vi "DataTranslation_server.vi"(0 "Board type":T1=enum."DT LV-link", 1 "interval scanning":bool, 2 "Client Time":dbl=3399992102.447224, 5 "No of samples+extra":i32=200 min=0 step=1, 7 "Trigger mode":T2, 9 "output polarity":u16(ring)=1 items=["do not change", "positive", "negative"], 11 "Ch & spans":T3[](array[typedef])=[{"high limit (10V)"=10.0, "low limit (-10V)"=-10.0, "Ch No"=0, "Var name"="RV (Vin)", "Use Latest Calib"=FALSE}] {"low limit (-10V)" format="%.3f"; "high limit (10V)" format="%.3f"}, 12 "Actual Sampling rate (Hz)":dbl=10000.0 format="%.2f", 13 "Local Client?":bool=TRUE, 14 "Current Block No":i32) -> (4 "I16 data":i16[][](array[numeric]), 6 "Block Timings":T4={"Started"=3399991568.753699, "Ended"=3399991587.0837474, "Analogue Frequency Hz"=50000.0} {"Analogue Frequency Hz" format="%.2f"}, 10 "group channel settings":T5(array[cluster])=[{"channel"="", "upper input limits"=0.0, "lower input limits"=0.0, "range"=0.0, "polarity"=0, "gain"=0.0, "coupling"=0, "input mode"=0, "scale multiplier"=1.6666666666666668e-07, "scale offset"=0.0}] {"scale offset" format="%#_16f"; "scale multiplier" format="%#_16f"; "input mode" format="%#_16f"; "coupling" format="%#_16f"; "gain" format="%#_16f"; "polarity" format="%#_16f"; "range" format="%#_16f"; "lower input limits" format="%#_16f"; "upper input limits" format="%#_16f"}, 15 "error out":errorcluster={"status"=TRUE, "code"=1172, "source"="Error calling method LvLink2.LvTask.ReadDblData2DAs1D, (System.Reflection.TargetInvocationException: Exception has been thrown by the target of an invocation.\n\tInner Exception: LvLink2.LvException: Timeout) <append><b>LvLink2.LvException</b> in OLReadMultiple2D.vi->DataTranslation_server.vi->Acquire_Data.vi->Get_data.vi->Measurement.vi"})   [LabVIEW 2011]
uses:
  Controls/Block_start_and_end.ctl
  Data_Translation/DataTranslation_global.vi
  Globals/Meas_global.vi
  <userlib>/LV-Link3/PolySubVIs/DtCreateAinChan.vi
  PWA/PWAtasksGLOBAL.vi
  <userlib>/LV-Link3/PolySubVIs/DtOLTimingSetInput.vi
  <userlib>/LV-Link3/PolySubVIs/DtOLReadMultiple2D.vi
  <userlib>/LV-Link3/PolySubVIs/DtOLTriggerDigital.vi
  Controls/Ch_and_Spans.ctl
  Controls/Trigger_Mode.ctl
  Controls/Board_Types.ctl
panel:
  in  "error in":errorcluster
  out "AFG error out":errorcluster
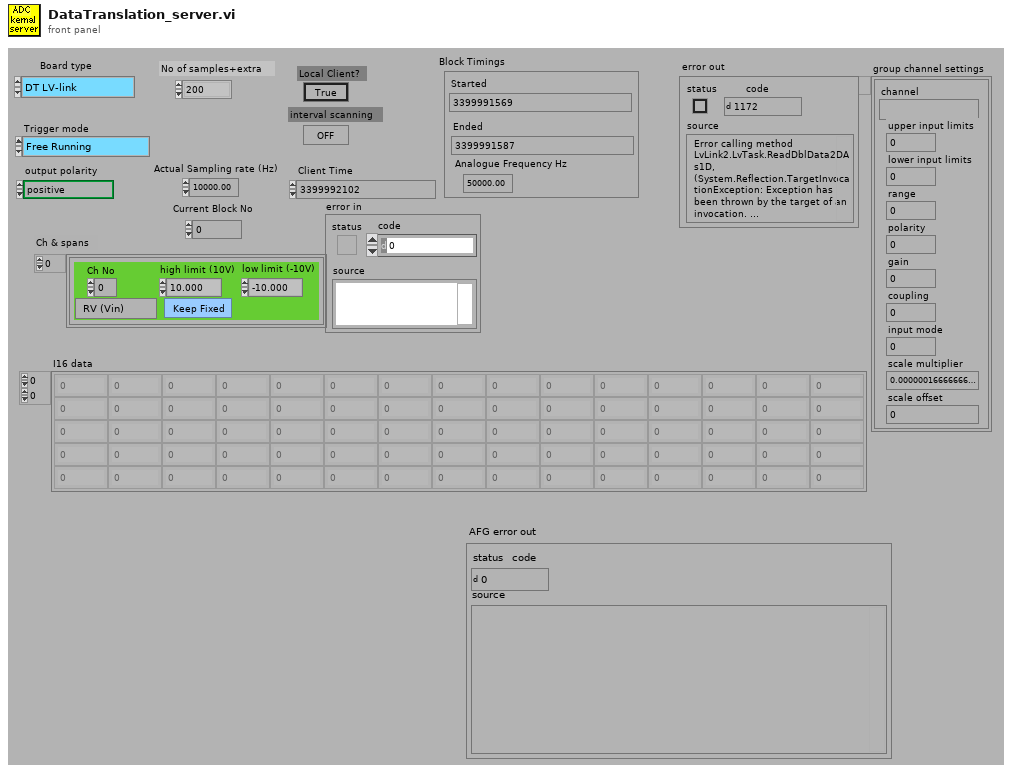
[diagram p1: front panel]
types:
  T1 = typedef "Board_Types.ctl" = enum16{"Simulate", "Local ADAM", "Server ADAM", "NI-DAQmx", "NI-DAQmxBase", "ADC488", "DT LV-link"}
  T2 = typedef "Trigger_Mode.ctl" = enum16{"Free Running", "Start on Trigger", "Trigger Every Block", "Trigger Every Sample"}
  T3 = typedef "Ch_and_Spans.ctl" = cluster{"high limit (10V)":sgl, "low limit (-10V)":sgl, "Ch No":i16, "Var name":string, "Use Latest Calib":bool}
  T4 = typedef "Block_start_and_end.ctl" = cluster{"Started":dbl, "Ended":dbl, "Analogue Frequency Hz":dbl}
  T5 = cluster{"channel":string, "upper input limits":sgl, "lower input limits":sgl, "range":sgl, "polarity":u16, "gain":sgl, "coupling":u16, "input mode":u16, "scale multiplier":dbl, "scale offset":dbl}[]
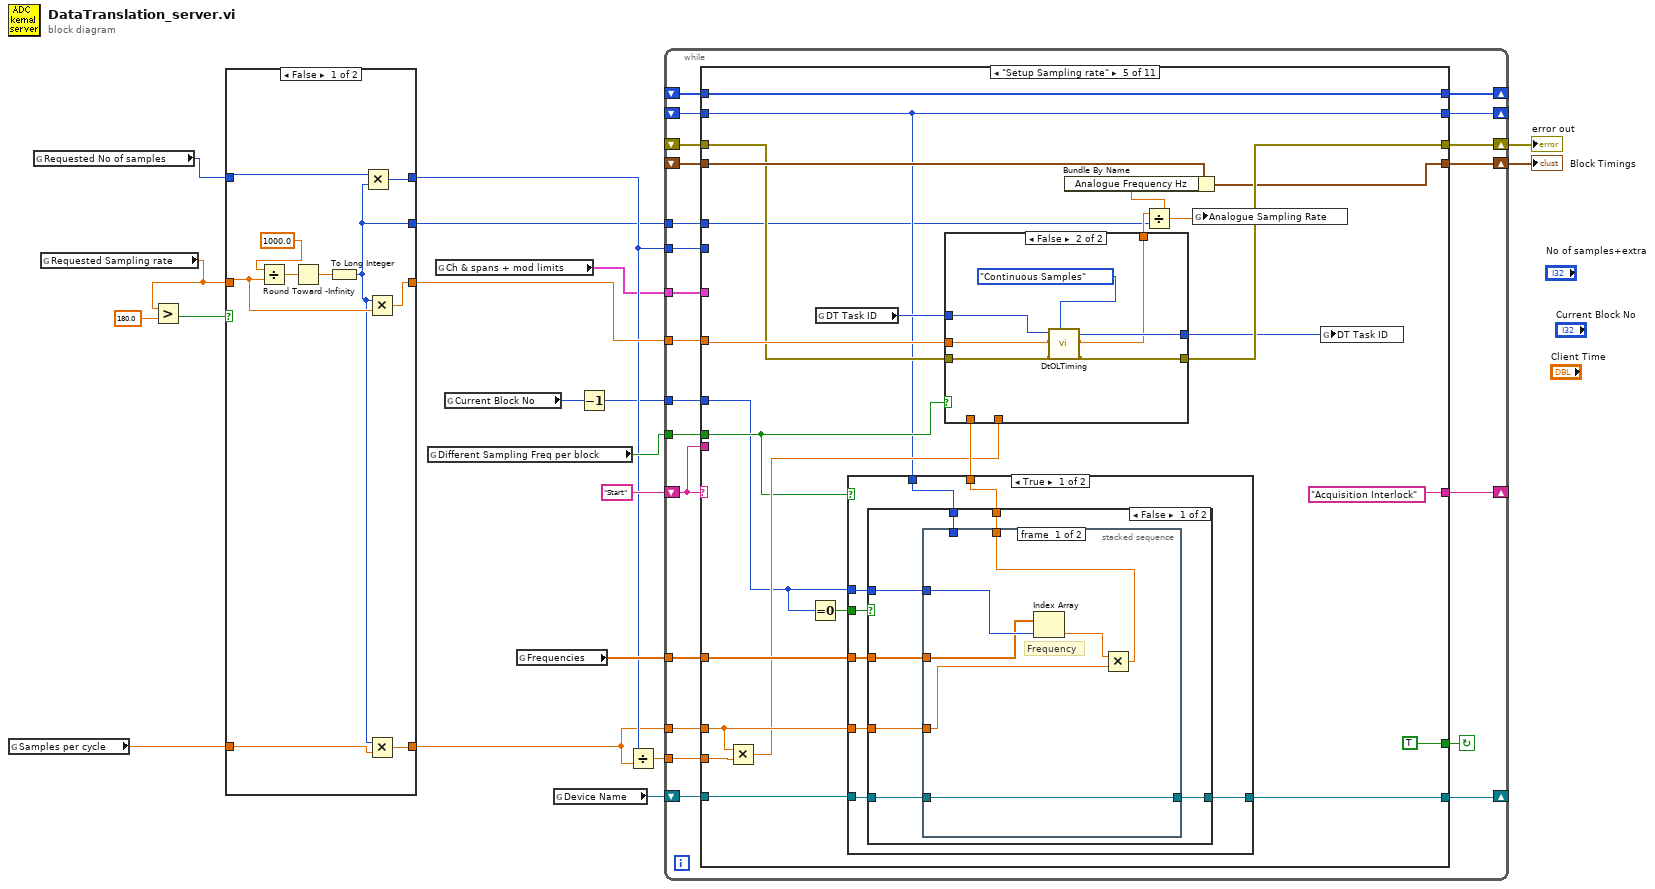
[diagram p0: block diagram]
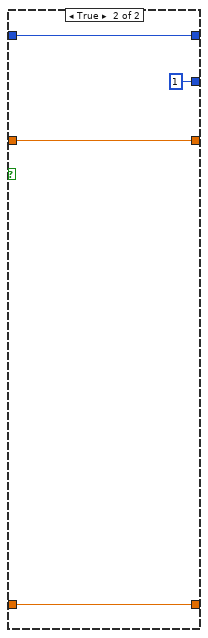
[diagram p2: hidden frame]
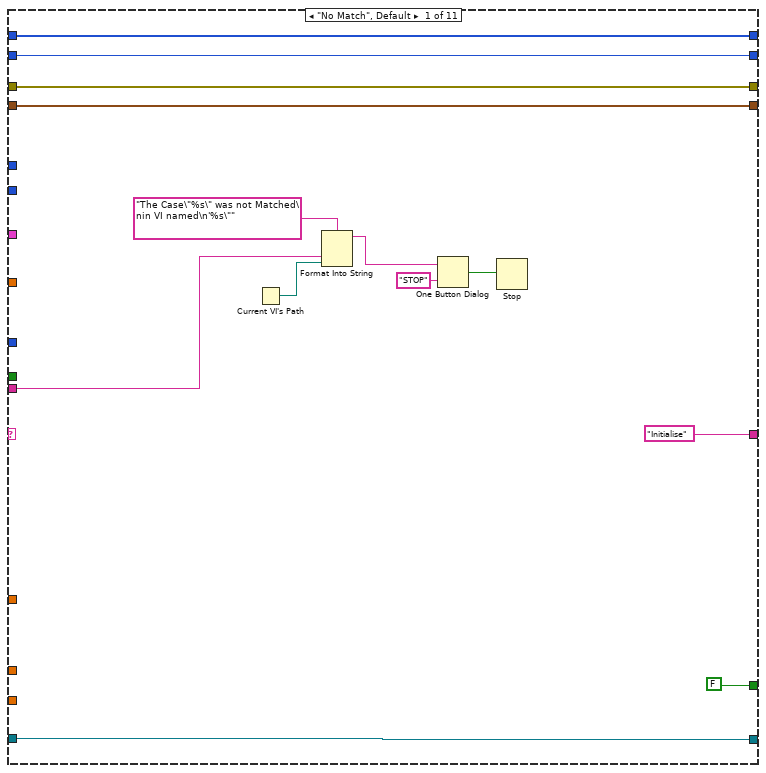
[diagram p3: hidden frame]
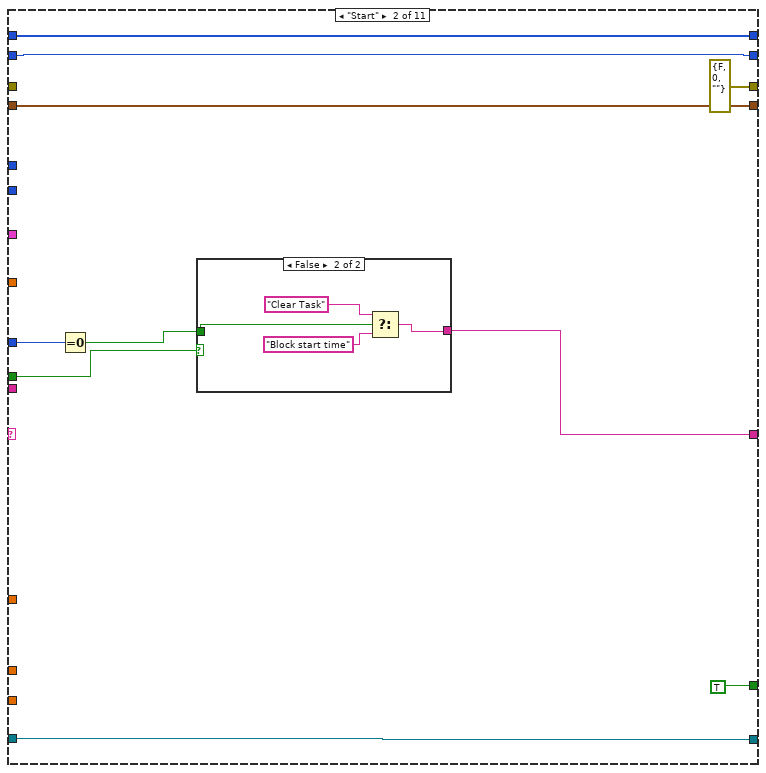
[diagram p4: hidden frame]
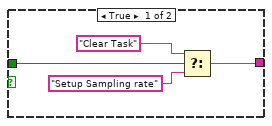
[diagram p5: hidden frame]
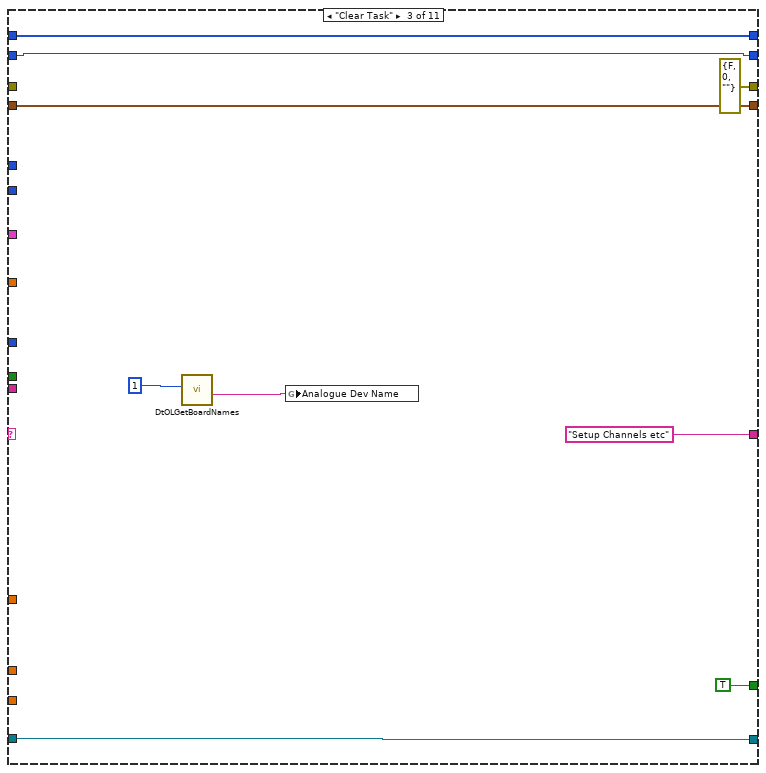
[diagram p6: hidden frame]
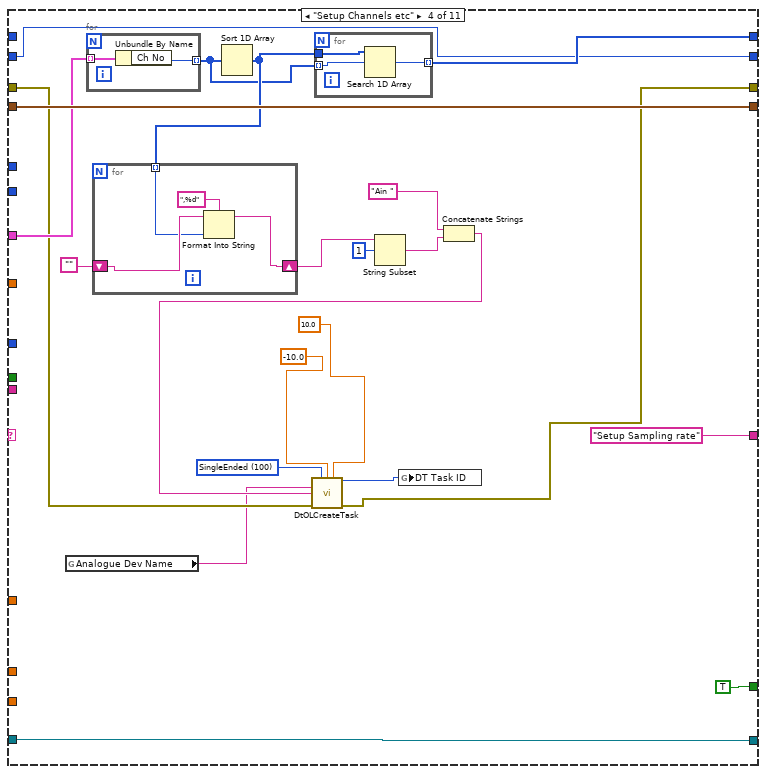
[diagram p7: hidden frame]
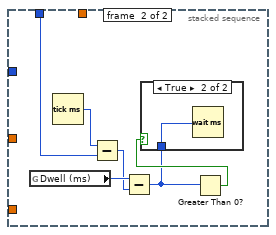
[diagram p8: hidden frame]
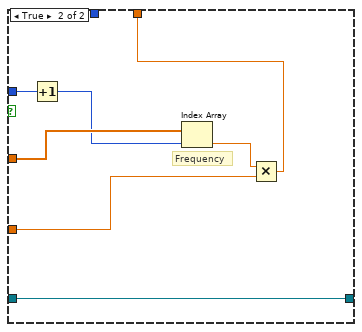
[diagram p10: hidden frame]
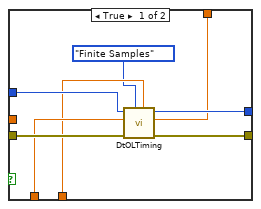
[diagram p12: hidden frame]
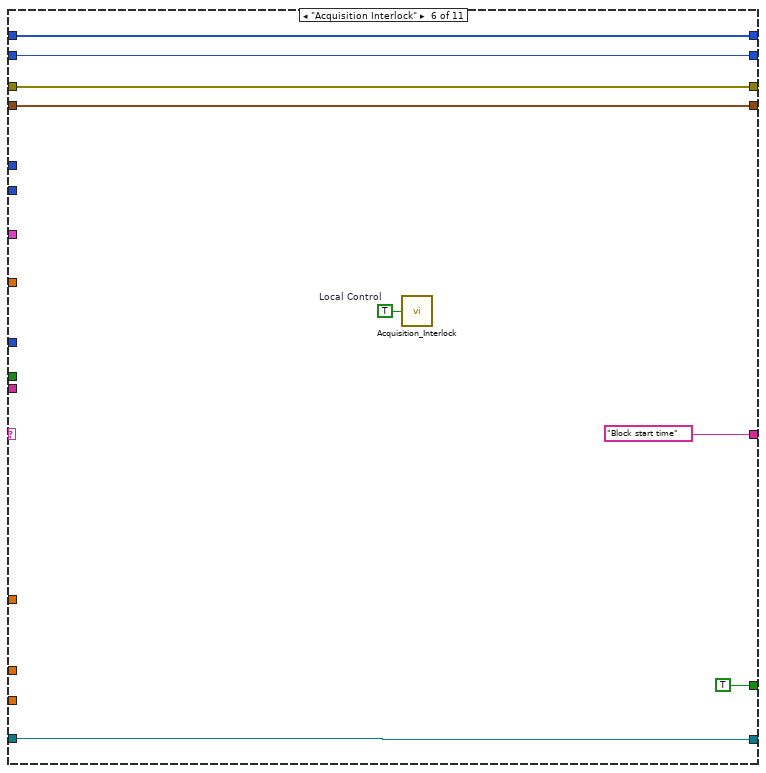
[diagram p13: hidden frame]
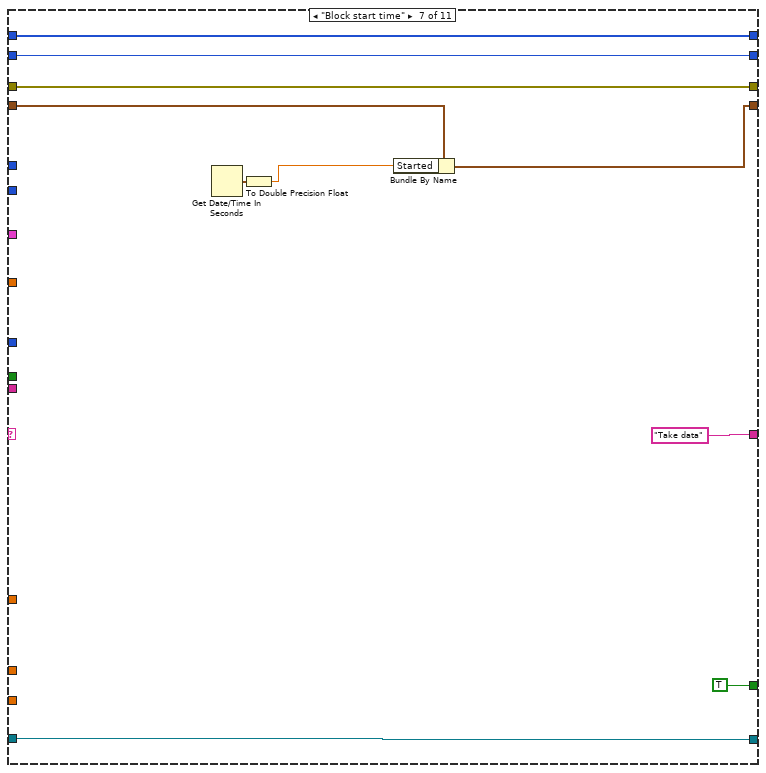
[diagram p14: hidden frame]
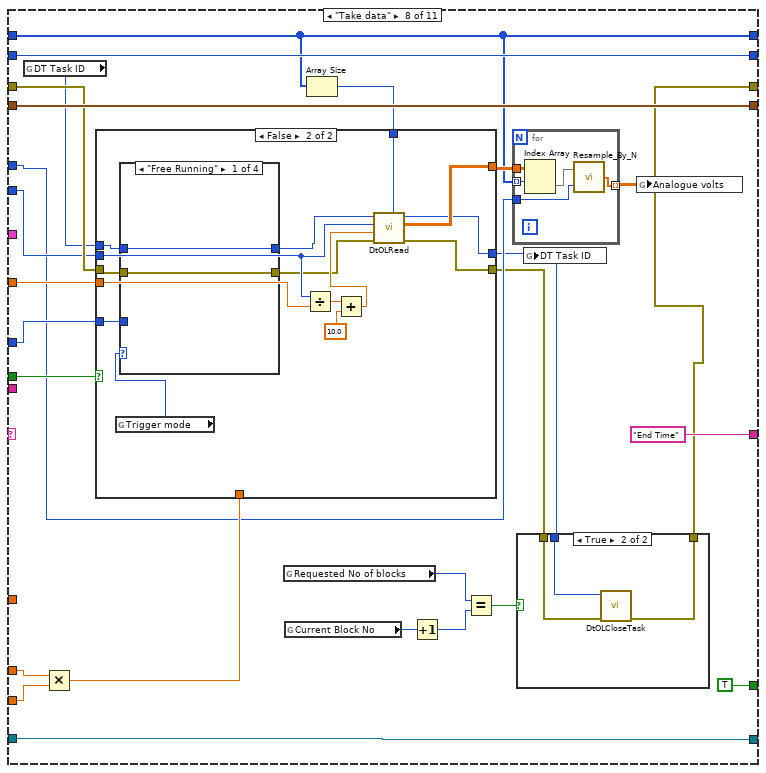
[diagram p15: hidden frame]
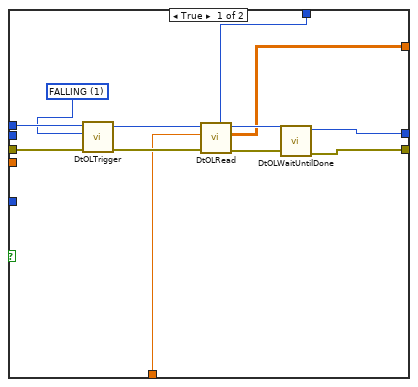
[diagram p17: hidden frame]
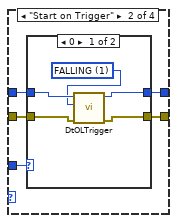
[diagram p18: hidden frame]
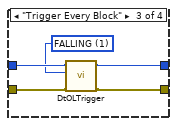
[diagram p20: hidden frame]
diagram:
  n1 = global read "DataTranslation_global.vi" "Samples per cycle"() -> (w7:dbl)
  n2 = global read "Meas_global.vi" "Requested No of samples"() -> (w1:i32)
  n3 = global read "Meas_global.vi" "Requested Sampling rate"() -> (w4:dbl)
  n4 = Greater?(x=w4, y=180.0) -> (0:w11:bool)
  n5 = case shown="False" w11 {
    tunnel: w4 -> [w23 w33]
    tunnel: [w24 w33] -> w10
    tunnel: [w26 w32] -> w9
    tunnel: w1 -> [w25 w32]
    tunnel: [w22 w31] -> w8
    tunnel: w7 -> [w21 w31]
    tunnel: [w20 1] -> w6
    frame False {
      n6 = Divide(x=1000.0, y=w23) -> (x/y=w28:dbl)
      n7 = Round Toward -Infinity(1:w28) -> (0:w27:dbl)
      n8 = To Long Integer(number=w27) -> (32bit integer=w20:i32)
      n9 = Multiply(x=w25, y=w20) -> (x*y=w26:i32)
      n10 = Multiply(x=w20, y=w23) -> (x*y=w24:dbl)
      n11 = Multiply(x=w20, y=w21) -> (x*y=w22:dbl)
    }
    frame True {
    }
  }
  n12 = global read "DataTranslation_global.vi" "Different Sampling Freq per block"() -> (w13:bool)
  n13 = global read "Meas_global.vi" "Ch & spans + mod limits"() -> (w5:T3[])
  n14 = global read "Meas_global.vi" "Current Block No"() -> (w3:i32)
  n15 = global read "DataTranslation_global.vi" "Frequencies"() -> (w14:dbl[])
  n16 = global read "DataTranslation_global.vi" "Device Name"() -> (w15:refnum<visa-resource-name>)
  n17 = Decrement(x=w3) -> (x-1=w2:i32)
  n18 = Divide(x=w9, y=w8) -> (x/y=w16:dbl)
  n19 = while {
    shift-left: "Start" -> [w53]
    shift-right: [w54] -> _
    shift-right: [w46] -> w17
    shift-left: _ -> [w52]
    shift-right: [w45] -> w18
    shift-left: _ -> [w51]
    tunnel: w10 -> [w50]
    tunnel: w9 -> [w49]
    tunnel: w2 -> [w48]
    tunnel: w5 -> [w47]
    shift-right: [w44] -> _
    shift-left: _ -> [w43]
    tunnel: w8 -> [w41]
    shift-right: [w40] -> _
    shift-left: w15 -> [w42]
    tunnel: w16 -> [w39]
    tunnel: w13 -> [w38]
    tunnel: w14 -> [w37]
    shift-right: [w36] -> _
    shift-left: _ -> [w35]
    tunnel: w6 -> [w34]
    stop <- w55 continue-if-true
    n20 = case shown="\"Setup Sampling rate\"" w53 {
      tunnel: [FALSE TRUE TRUE TRUE TRUE TRUE TRUE TRUE w307 FALSE FALSE] -> w55
      tunnel: ["Initialise" w74 "Setup Channels etc" "Setup Sampling rate" "Acquisition Interlock" "Block start time" "Take data" "End Time" "Add info to block header" ("f") "End" ("f") "End" ("f")] -> w54
      tunnel: w53 -> [w63 _ _ _ _ _ _ _ _ _ _]
      tunnel: [w60 errorcluster {"status"=FALSE, "code"=0, "source"=""} ("error out") errorcluster {"status"=FALSE, "code"=0, "source"=""} ("error out") w98 w149 w209 w217 w222 w309 w329 w374] -> w46
      tunnel: w52 -> [w60 _ _ w99 w145 w209 w217 w243 w309 w329 w374]
      tunnel: [w59 w77 w94 w110 w146 w207 w218 w244 w311 w327 T4 {"Started"=0.0, "Ended"=0.0, "Analogue Frequency Hz"=1000.0} ("Block Timings")] -> w45
      tunnel: w51 -> [w59 w77 w94 w110 w147 w207 w219 w244 w312 w327 _]
      tunnel: w50 -> [_ _ _ _ w148 _ _ w239 _ _ _]
      tunnel: w49 -> [_ _ _ _ _ _ _ w240 _ _ _]
      tunnel: w48 -> [_ w76 _ _ w131 _ _ w232 _ w317 _]
      tunnel: w47 -> [_ _ _ w109 _ _ _ _ _ _ _]
      tunnel: [w58 w72 w92 w106 w142 w206 w214 w231 w308 w328 w372] -> w44
      tunnel: w43 -> [w58 w72 w92 _ w142 w206 w214 w231 w308 w328 w372]
      tunnel: w42 -> [w57 w71 w91 w105 w139 w205 w213 w238 w306 w326 w371]
      tunnel: w37 -> [_ _ _ _ w141 _ _ _ _ w322 _]
      tunnel: w41 -> [_ _ _ _ w135 _ _ w236 _ _ _]
      tunnel: [w57 w71 w91 w105 w138 w205 w213 w238 w306 w325 w371] -> w40
      tunnel: w39 -> [_ _ _ _ w136 _ _ w237 _ _ _]
      tunnel: w38 -> [_ w70 _ _ w133 _ _ w234 w307 _ _]
      tunnel: [w56 w69 w90 w104 w132 w204 w212 w233 w305 w319 w370] -> w36
      tunnel: w35 -> [w56 w69 w90 w104 w132 w204 w212 w233 w305 _ w370]
      tunnel: w34 -> [_ _ _ _ w128 _ _ w229 _ _ _]
      frame "No Match", Default {
        n21 = Current VI's Path() -> (path=w62:path)
        n22 = Format Into String(format string="The Case\"%s\" was not Matched\nin VI named\n'%s\"" ("Format String"), w63, w62) -> (resulting string=w66:string)  [unwired: 2 in, 1 out]
        n23 = One Button Dialog(message=w66, button name ("OK")="STOP") -> (true=w64:bool)
        n24 = Stop(stop? (T)=w64) -> ()
      }
      frame "Start" {
        n25 = Equal To 0?(x=w76) -> (x = 0?=w75:bool)
        n26 = case shown="False" w70 {
          tunnel: w75 -> [w80 w84]
          tunnel: [w79 w83] -> w74
          frame True {
            n27 = Select(t="Clear Task", s=w80, f="Setup Sampling rate") -> (s? t:f=w79:string)
          }
          frame False {
            n28 = Select(t="Clear Task", s=w84, f="Block start time") -> (s? t:f=w83:string)
          }
        }
      }
      frame "Clear Task" {
        n29 = call <userlib>:"DtOLGetBoardNames.vi"("Select Board"=u32 1) -> ("Board Name"=w88:string)  [unwired: 8 in, 2 out]
        n30 = global write "PWAtasksGLOBAL.vi" "Analogue Dev Name"(w88) -> ()
      }
      frame "Setup Channels etc" {
        w100 = 100 items=["SingleEnded"=100, "Differential"=101] ("Channel Type")
        n31 = global read "PWAtasksGLOBAL.vi" "Analogue Dev Name"() -> (w96:string)
        n32 = for {
          tunnel: w109 -> [w122] mode=indexing
          tunnel: [w121] -> w107 mode=indexing
          n33 = Unbundle By Name(w122) -> ("Ch No"=w121:i16)
        }
        n34 = Sort 1D Array(array=w107) -> (sorted array=w108:i16[])
        n35 = for {
          shift-right: [w124] -> w115
          shift-left: "" -> [w125]
          tunnel: w108 -> [w123] mode=indexing
          n36 = Format Into String(format string=",%d", initial string=w125, w123) -> (resulting string=w124:string)  [unwired: 1 in, 1 out]
        }
        n37 = for {
          tunnel: w108 -> [w120]
          tunnel: w107 -> [w119] mode=indexing
          tunnel: [w118] -> w106 mode=indexing
          n38 = Search 1D Array(1D array=w120, element=w119) -> (index of element=w118:i32)  [unwired: 1 in]
        }
        n39 = String Subset(string=w115, offset (0)=1) -> (substring=w112:string)  [unwired: 1 in]
        n40 = Concatenate Strings("Ain ", w112) -> (w103:string)
        n41 = call-poly <userlib>:"DtOLCreateTask.vi"("Channel Type"=w100, "Range Min"=-10.0, "Range Max"=10.0, "Board Name"=w96, "Channel"=w103, "error in (no error)"=w99) -> ("Task out"=w97:i32, "error out"=w98:errorcluster)  [unwired: 7 in, 1 out]
        n42 = global write "DataTranslation_global.vi" "DT Task ID"(w97) -> ()
      }
      frame "Setup Sampling rate" {
        n43 = Multiply(x=w135, y=w136) -> (x*y=w134:dbl)
        n44 = Equal To 0?(x=w131) -> (x = 0?=w130:bool)
        n45 = global read "DataTranslation_global.vi" "DT Task ID"() -> (w143:i32)
        n46 = case shown="True" w133 {
          tunnel: w141 -> [w154 _]
          tunnel: [w158 w186] -> w140
          tunnel: w135 -> [w157 w186]
          tunnel: w131 -> [w156 _]
          tunnel: w139 -> [w155 w187]
          tunnel: [w153 w187] -> w138
          tunnel: w132 -> [w152 _]
          tunnel: w130 -> [w151 _]
          frame True {
            n47 = case shown="False" w151 {
              tunnel: [w165 w182] -> w158
              tunnel: w157 -> [w164 w181]
              tunnel: w156 -> [w159 w183]
              tunnel: w155 -> [w163 w180]
              tunnel: w154 -> [w162 w184]
              tunnel: [w161 w180] -> w153
              tunnel: w152 -> [w160 _]
              frame False {
                n48 = stacked-sequence {
                  tunnel: [w171 _] -> w165
                  tunnel: w164 -> [w170 _]
                  tunnel: w159 -> [w169 _]
                  tunnel: w163 -> [w166 _]
                  tunnel: w162 -> [w168 _]
                  tunnel: [w166 _] -> w161
                  tunnel: w160 -> [_ w176]
                  frame #0 {
                    # "Frequency"
                    n49 = Index Array(array=w168, index=w169) -> (element=w167:dbl)
                    n50 = Multiply(x=w167, y=w170) -> (x*y=w171:dbl)
                  }
                  frame #1 {
                    n51 = global read "DataTranslation_global.vi" "Dwell (ms)"() -> (w175:u32)
                    n52 = Tick Count (ms)() -> (millisecond timer value=w177:u32)
                    n53 = Subtract(x=w177, y=w176) -> (x-y=w174:u32)
                    n54 = Subtract(x=w175, y=w174) -> (x-y=w172:u32)
                    n55 = Greater Than 0?(x=w172) -> (x > 0?=w173:bool)
                    n56 = case shown="True" w173 {
                      tunnel: w172 -> [_ w178]
                      frame False {
                      }
                      frame True {
                        n57 = Wait (ms)(milliseconds to wait=w178) -> ()  [unwired: 1 out]
                      }
                    }
                  }
                }
              }
              frame True {
                # "Frequency"
                n58 = Increment(x=w183) -> (x+1=w179:i32)
                n59 = Index Array(array=w184, index=w179) -> (element=w185:dbl)
                n60 = Multiply(x=w185, y=w181) -> (x*y=w182:dbl)
              }
            }
          }
          frame False {
          }
        }
        n61 = case shown="False" w133 {
          tunnel: [w192 w197] -> w149
          tunnel: w148 -> [_ w200]
          tunnel: [w191 w199] -> w129
          tunnel: w145 -> [w193 w198]
          tunnel: [w194 w202] -> w144
          tunnel: w143 -> [w195 w201]
          tunnel: w140 -> [w190 _]
          tunnel: w134 -> [w189 _]
          frame True {
            n62 = call-poly <userlib>:"DtOLTiming.vi"("Samples Per Channel"=w189, "Sample Mode"=enum16{"Finite Samples", "Continuous Samples"}."Finite Samples", "error in (no error)"=w193, "Sample Freq (Hz)"=w190, "Task in"=w195) -> ("error out"=w192:errorcluster, "Actual Sample Freq"=w191:dbl, "Task out"=w194:i32)  [unwired: 3 in, 1 out]
          }
          frame False {
            n63 = call-poly <userlib>:"DtOLTiming.vi"("Sample Mode"=enum16{"Finite Samples", "Continuous Samples"}."Continuous Samples", "error in (no error)"=w198, "Sample Freq (Hz)"=w200, "Task in"=w201) -> ("error out"=w197:errorcluster, "Actual Sample Freq"=w199:dbl, "Task out"=w202:i32)  [unwired: 4 in, 1 out]
          }
        }
        n64 = Divide(x=w129, y=w128) -> (x/y=w127:dbl)
        n65 = Bundle By Name(cluster=w147, "Analogue Frequency Hz"=w127) -> (w146:T4)
        n66 = global write "Meas_global.vi" "Analogue Sampling Rate"(w127) -> ()
        n67 = global write "DataTranslation_global.vi" "DT Task ID"(w144) -> ()
      }
      frame "Acquisition Interlock" {
        w203 = TRUE  # Local Control
        n68 = call "Acquisition_Interlock.vi"("Local Control"=w203) -> ()
      }
      frame "Block start time" {
        n69 = Get Date/Time In Seconds() -> (seconds since 1Jan1904=w220:timestamp)
        n70 = To Double Precision Float(number=w220) -> (double precision float=w211:dbl)
        n71 = Bundle By Name(cluster=w219, "Started"=w211) -> (w218:T4)
      }
      frame "Take data" {
        n72 = global read "DataTranslation_global.vi" "DT Task ID"() -> (w242:i32)
        n73 = Multiply(x=w236, y=w237) -> (x*y=w235:dbl)
        n74 = global read "Meas_global.vi" "Requested No of blocks"() -> (w226:i32)
        n75 = global read "Meas_global.vi" "Current Block No"() -> (w228:i32)
        n76 = Array Size(array=w231) -> (size(s)=w230:i32)
        n77 = case shown="False" w234 {
          tunnel: w243 -> [w262 w272]
          tunnel: [w259 w266] -> w223
          tunnel: [w256 w264] -> w225
          tunnel: w242 -> [w255 w273]
          tunnel: [w253 w265] -> w241
          tunnel: w240 -> [_ w269]
          tunnel: w239 -> [_ w277]
          tunnel: w235 -> [w252 _]
          tunnel: w232 -> [_ w271]
          tunnel: w230 -> [w251 w263]
          frame True {
            w254 = 1 items=["RISING", "FALLING"] ("External Trigger Polarity")
            n78 = call-poly <userlib>:"DtOLTrigger.vi"("error in (no error)"=w262, "External Trigger Polarity"=w254, "Task in"=w255) -> ("error out"=w261:errorcluster, "Task out"=w258:i32)  [unwired: 7 in]
            n79 = call-poly <userlib>:"DtOLRead.vi"("Number Chan to Read"=w251, "error in (no error)"=w261, "Samples Per Channel"=w252, "Task in"=w258) -> ("error out"=w260:errorcluster, "2D Data out"=w253:dbl[][], "Task out"=w257:i32)  [unwired: 3 in, 2 out]
            n80 = call <userlib>:"DtOLWaitUntilDone.vi"("error in"=w260, "Task in"=w257) -> ("error out"=w259:errorcluster, "Task out"=w256:i32)  [unwired: 8 in]
          }
          frame False {
            n81 = global read "Meas_global.vi" "Trigger mode"() -> (w274:T2)
            n82 = case shown="\"Free Running\"" w274 {
              tunnel: [w279 w281 w295 w298] -> w270
              tunnel: w273 -> [w279 w283 w296 w298]
              tunnel: [w278 w280 w292 w297] -> w267
              tunnel: w272 -> [w278 w282 w293 w297]
              tunnel: w271 -> [_ w284 _ _]
              frame "Free Running" {
              }
              frame "Start on Trigger" {
                n83 = case shown="0" w284 {
                  tunnel: w283 -> [w289 w291]
                  tunnel: w282 -> [w287 w290]
                  tunnel: [w285 w291] -> w281
                  tunnel: [w286 w290] -> w280
                  frame 0 {
                    w288 = 1 items=["RISING", "FALLING"] ("External Trigger Polarity")
                    n84 = call-poly <userlib>:"DtOLTrigger.vi"("error in (no error)"=w287, "External Trigger Polarity"=w288, "Task in"=w289) -> ("error out"=w286:errorcluster, "Task out"=w285:i32)  [unwired: 7 in]
                  }
                  frame 1, Default {
                  }
                }
              }
              frame "Trigger Every Block" {
                w294 = 1 items=["RISING", "FALLING"] ("External Trigger Polarity")
                n85 = call-poly <userlib>:"DtOLTrigger.vi"("error in (no error)"=w293, "External Trigger Polarity"=w294, "Task in"=w296) -> ("error out"=w292:errorcluster, "Task out"=w295:i32)  [unwired: 7 in]
              }
              frame "Trigger Every Sample" {
              }
            }
            n86 = Divide(x=w269, y=w277) -> (x/y=w275:dbl)
            n87 = Add(x=w275, y=10.0) -> (x+y=w268:dbl)
            n88 = call-poly <userlib>:"DtOLRead.vi"("Number Chan to Read"=w263, "error in (no error)"=w267, "Timeout"=w268, "Samples Per Channel"=w269, "Task in"=w270) -> ("error out"=w266:errorcluster, "2D Data out"=w265:dbl[][], "Task out"=w264:i32)  [unwired: 2 in, 2 out]
          }
        }
        n89 = Increment(x=w228) -> (x+1=w227:i32)
        n90 = Equal?(x=w226, y=w227) -> (x = y?=w224:bool)
        n91 = for {
          tunnel: w231 -> [w303] mode=indexing
          tunnel: w241 -> [w302]
          tunnel: [w300] -> w221 mode=indexing
          tunnel: w229 -> [w299]
          n92 = Index Array(array=w302, index (row)=w303) -> (element=w301:dbl[])  [unwired: 1 in]
          n93 = call "Resample_By_N.vi"("Resample Factor"=w299, "Array In"=w301) -> ("Array Out"=w300:dbl[])
        }
        n94 = case shown="True" w224 {
          tunnel: w225 -> [_ w250]
          tunnel: w223 -> [w247 w249]
          tunnel: [w247 w248] -> w222
          frame False {
          }
          frame True {
            n95 = call <userlib>:"DtOLCloseTask.vi"("Error in"=w249, "Task in"=w250) -> ("Error Out"=w248:errorcluster)  [unwired: 9 in]
          }
        }
        n96 = global write "DataTranslation_global.vi" "DT Task ID"(w225) -> ()
        n97 = global write "Meas_global.vi" "Analogue volts"(w221) -> ()
      }
      frame "End Time" {
        # "Final transpose to get 2D data output correctly"
        n98 = Get Date/Time In Seconds() -> (seconds since 1Jan1904=w313:timestamp)
        n99 = To Double Precision Float(number=w313) -> (double precision float=w304:dbl)
        n100 = Bundle By Name(cluster=w312, "Ended"=w304) -> (w311:T4)
      }
      frame "Add info to block header" {
        n101 = global read "Meas_global.vi" "Requested No of blocks"() -> (w320:i32)
        n102 = global read "DataTranslation_global.vi" "Amplitudes"() -> (w314:dbl[])
        n103 = Index Array(array=w314, index=w317) -> (element=w324:dbl)
        n104 = Index Array(array=w322, index=w317) -> (element=w323:dbl)
        n105 = Decrement(x=w320) -> (x-1=w318:i32)
        n106 = for {
          tunnel: [w359] -> _ mode=indexing
          tunnel: w324 -> [w358]
          tunnel: w323 -> [w357]
          i -> [w360]
          n107 = case shown="0" w360 {
            tunnel: [w364 _] -> w359
            tunnel: w358 -> [w367 _]
            tunnel: w357 -> [w366 _]
            frame 0 {
              n108 = call "Value_to_string.vi"("Value"=w367, "Label for value"="Function_Generator_Amplitude") -> ("Output string"=w363:string)  [unwired: 1 in]
              n109 = call "Value_to_string.vi"("precision"="0", "Value"=w366, "Label for value"="Function_Generator_Frequency") -> ("Output string"=w362:string)
              n110 = Concatenate Strings(w363, w362) -> (w361:string)
              n111 = Bundle By Name("channel"=w361) -> (w364:cluster{})  [unwired: 1 in]
            }
            frame 1, Default {
            }
          }
        }
        n112 = Equal?(x=w317, y=w318) -> (x = y?=w321:bool)
        n113 = case shown="False" w321 {
          tunnel: w326 -> [w344 w354]
          tunnel: [w335 w352] -> w325
          tunnel: [w337 w353] -> w315
          tunnel: w322 -> [w340 w355]
          tunnel: w314 -> [w341 w356]
          tunnel: w317 -> [w339 _]
          tunnel: [w341 w356] -> _
          tunnel: [w340 w355] -> _
          tunnel: "error in" -> [w332 w350]
          frame False {
            w345 = "SOUR1" ("input 1")
            w348 = ":%s:FREQ %.;%g;"  # Frequency Command
            w349 = ":%s:VOLT %.;%g;"  # Amplitude Command
            n114 = Increment(x=w339) -> (x+1=w338:i32)
            n115 = Index Array(array=w341, index=w338) -> (element=w343:dbl)
            n116 = Index Array(array=w340, index=w338) -> (element=w342:dbl)
            n117 = Format Into String(format string=w348, w345, w342) -> (resulting string=w346:string)  [unwired: 2 in, 1 out]
            n118 = Format Into String(format string=w349, initial string=w346, w345, w343) -> (resulting string=w347:string)  [unwired: 1 in, 1 out]
            n119 = VISA Write(VISA resource name=w344, write buffer=w347, error in (no error)=w332) -> (VISA resource name out=w336:refnum<visa-resource-name>, error out=w334:errorcluster)  [unwired: 1 out]
            n120 = VISA Write(VISA resource name=w336, write buffer="OUTP1:STAT ON", error in (no error)=w334) -> (VISA resource name out=w335:refnum<visa-resource-name>, error out=w337:errorcluster)  [unwired: 1 out]
          }
          frame True {
            n121 = VISA Write(VISA resource name=w354, write buffer="OUTP1:STAT OFF", error in (no error)=w350) -> (VISA resource name out=w352:refnum<visa-resource-name>, error out=w353:errorcluster)  [unwired: 1 out]
          }
        }
        "AFG error out" <- w315
        n122 = Tick Count (ms)() -> (millisecond timer value=w319:u32)
      }
      frame "Extra case" {
      }
    }
  }
  "Block Timings" <- w18
  "error out" <- w17
